vi "BouncingBall.vi"() -> ()   [LabVIEW 2022 SP3]
uses:
  <vilib>/Utility/miscctls.llb/LVPositionTypeDef.ctl
panel:
  in  "stop":bool
  out "Top":bool
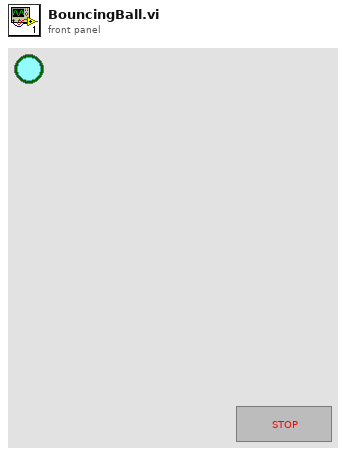
[diagram p1: front panel]
types:
  T1 = typedef "LVPositionTypeDef.ctl" = cluster{"Left":i32, "Top":i32}
  T2 = cluster{"Position":T1, "Step":T1, "BarPosition":T1}
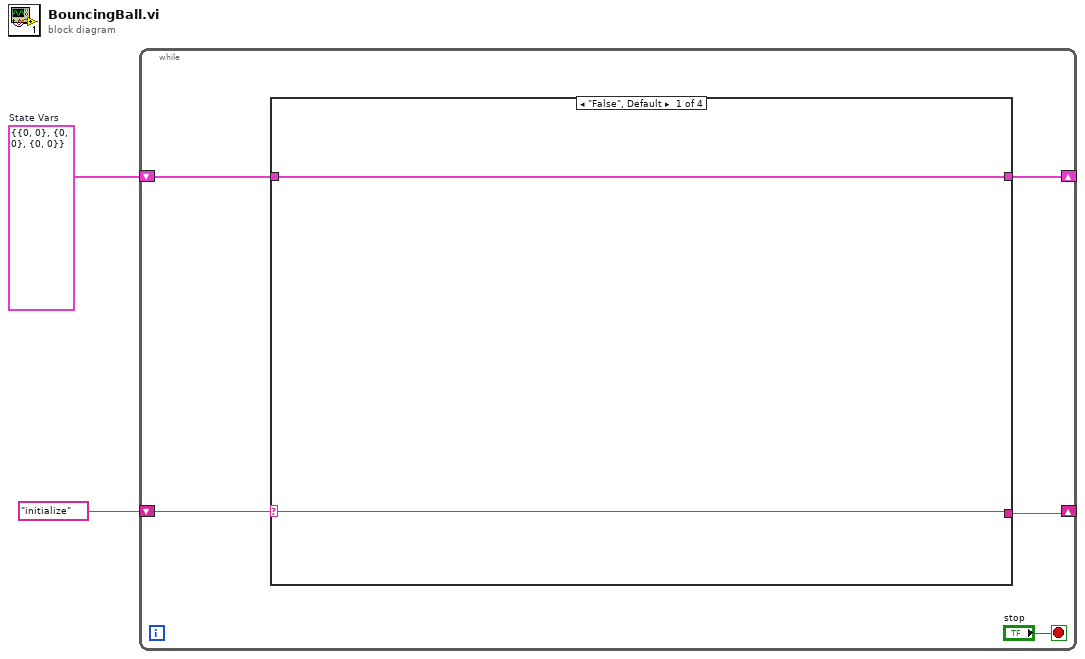
[diagram p0: block diagram]
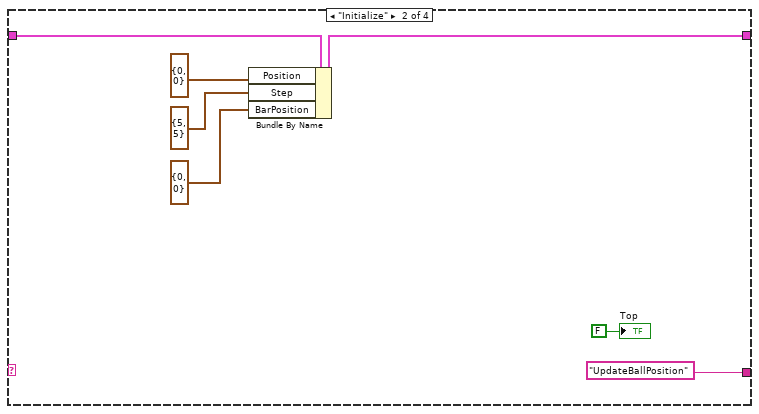
[diagram p2: hidden frame]
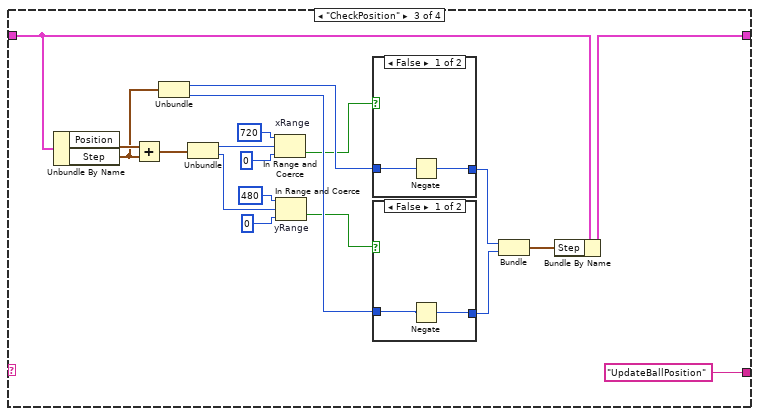
[diagram p3: hidden frame]
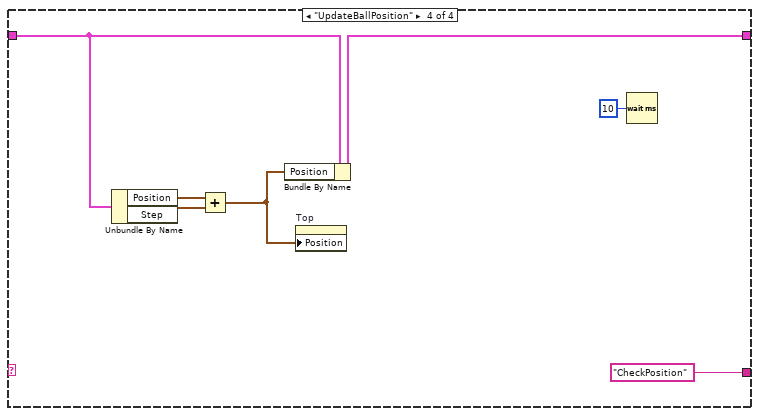
[diagram p6: hidden frame]
diagram:
  w1 = T2 {"Position"={"Left"=0, "Top"=0}, "Step"={"Left"=0, "Top"=0}, "BarPosition"={"Left"=0, "Top"=0}}  # State Vars
  n1 = while {
    shift-right: [w4] -> _
    shift-left: "initialize" -> [w3]
    shift-right: [w5] -> _
    shift-left: w1 -> [w6]
    stop <- "stop" stop-if-true
    n2 = case shown="\"False\", Default" w3 {
      selector: w3 -> [w8 _ _ _]
      tunnel: w6 -> [w9 w16 w35 w42]
      tunnel: [w9 w15 w19 w46] -> w5
      tunnel: [w8 "UpdateBallPosition" "UpdateBallPosition" "CheckPosition"] -> w4
      frame "False", Default {
      }
      frame "Initialize" {
        n3 = Bundle By Name(cluster=w16, "Position"=T1 {"Left"=0, "Top"=0}, "Step"=T1 {"Left"=5, "Top"=5}, "BarPosition"=T1 {"Left"=0, "Top"=0} ("Position")) -> (w15:T2)
        "Top" <- FALSE ("Top")
      }
      frame "CheckPosition" {
        n4 = Unbundle By Name(w35) -> ("Position"=w34:T1, "Step"=w26:T1)
        n5 = Add(x=w34, y=w26) -> (x+y=w33:T1)
        n6 = Unbundle(w26) -> ("Left"=w25:i32, "Top"=w24:i32)
        n7 = Unbundle(w33) -> ("Left"=w32:i32, "Top"=w27:i32)
        n8 = In Range and Coerce "xRange"(upper limit=720, x=w32, lower limit=0) -> (In Range?=w23:bool)  [unwired: 1 out]
        n9 = In Range and Coerce "yRange"(upper limit=480, x=w27, lower limit=0) -> (In Range?=w22:bool)  [unwired: 1 out]
        n10 = case shown="False" w23 {
          tunnel: [w40 w41] -> w21
          tunnel: w25 -> [w39 w41]
          frame False {
            n11 = Negate(x=w39) -> (-x=w40:i32)
          }
          frame True {
          }
        }
        n12 = case shown="False" w22 {
          tunnel: [w37 w38] -> w20
          tunnel: w24 -> [w36 w38]
          frame False {
            n13 = Negate(x=w36) -> (-x=w37:i32)
          }
          frame True {
          }
        }
        n14 = Bundle("Left"=w21, "Top"=w20) -> (w18:cluster{"Left":i32, "Top":i32})  [unwired: 1 in]
        n15 = Bundle By Name(cluster=w35, "Step"=w18) -> (w19:T2)
      }
      frame "UpdateBallPosition" {
        n16 = Unbundle By Name(w42) -> ("Position"=w47:T1, "Step"=w48:T1)
        n17 = Add(x=w47, y=w48) -> (x+y=w45:T1)
        n18 = Bundle By Name(cluster=w42, "Position"=w45) -> (w46:T2)
        n19 = property on="Top" class="Bool (strict)"("Position"=w45) -> ()  [unwired: 2 in, 2 out]
        n20 = Wait (ms)(milliseconds to wait=u32 10) -> ()  [unwired: 1 out]
      }
    }
  }
